vi "Enqueue (Single).vi"(6 "Priority Message? Array":bool, 7 "timeout in ms (-1)":i32=-1, 8 "error in (no error)":errorcluster, 9 "Message Data Array":variant, 10 "States":T2, 11 "Message Queue":T1) -> (0 "error out":errorcluster, 3 "Message Queue dub":T1)   [LabVIEW 2019, in "Template.lvlib"]
doc: "For a regular message, enqueue the message. For a priority message, enqueue it at the front of the queue."
uses:
  Template.lvlib
  State Name.ctl
  Support/Shared/TypeDefs/Message Queue Ref.ctl
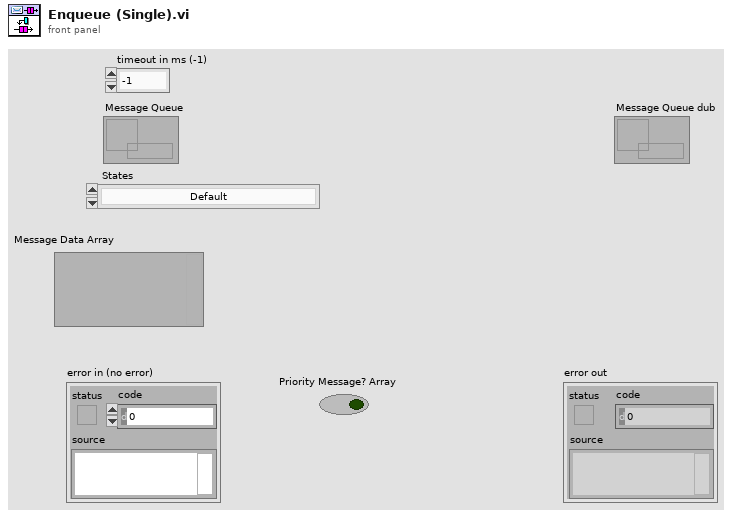
[diagram p1: front panel]
types:
  T1 = typedef "Message Queue Ref.ctl" = refnum<queue>
  T2 = typedef "Template.lvlib/State Name.ctl" = enum16{"Default", "Initialize", "Re-Initialize", "Initialize Data", "Initialize Panel", "[Event Structure] Update Data", "Error", "Exit"}
  T3 = cluster{string, "Variant":variant, string[], "Message Data Array":variant}
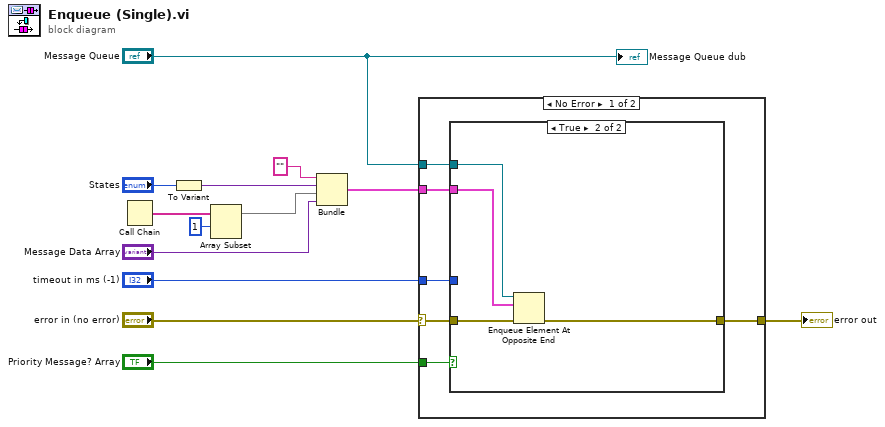
[diagram p0: block diagram]
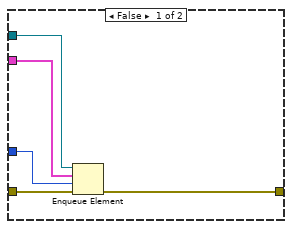
[diagram p2: hidden frame]
diagram:
  n1 = Call Chain() -> (call chain=w8:string[])
  n2 = To Variant(anything="States") -> (Variant=w6:variant)
  n3 = Array Subset(array=w8, index=1) -> (w2:string[])  [unwired: 1 in]
  n4 = Bundle("", "Variant"=w6, w2, "Message Data Array"="Message Data Array") -> (w4:T3)  [unwired: 1 in]
  n5 = case shown="No Error" "error in (no error)" {
    selector: "error in (no error)" -> [w14 w29]
    tunnel: "Priority Message? Array" -> [w19 _]
    tunnel: [w18 w29] -> w12
    tunnel: "Message Queue" -> [w17 _]
    tunnel: "timeout in ms (-1)" -> [w16 _]
    tunnel: w4 -> [w15 _]
    frame No Error {
      n6 = case shown="True" w19 {
        tunnel: w14 -> [w24 w28]
        tunnel: [w23 w27] -> w18
        tunnel: w17 -> [w22 w26]
        tunnel: w15 -> [w21 w25]
        tunnel: w16 -> [w20 _]
        frame False {
          n7 = Enqueue Element(queue=w22, element=w21, timeout in ms (-1)=w20, error in (no error)=w24) -> (error out=w23:errorcluster)  [unwired: 2 out]
        }
        frame True {
          n8 = Enqueue Element At Opposite End(queue=w26, element=w25, error in (no error)=w28) -> (error out=w27:errorcluster)  [unwired: 1 in, 2 out]
        }
      }
    }
    frame Error {
    }
  }
  "error out" <- w12
  "Message Queue dub" <- "Message Queue"
